vi "NIIE_Check whether installed.vi"(6 "Glyph Name":string, 9 "Glyph Pic":picture, 11 "Glyphs[]":T1[](array[typedef])) -> (1 "Image Out":picture, 2 "Match? Out":bool)   [LabVIEW 2021]
uses:
  MB CORE/TypeDefs/Cluster_Path&Icon.ctl
  vi.lib/LabVIEW Icon API/lv_icon/lv_icon.lvlib
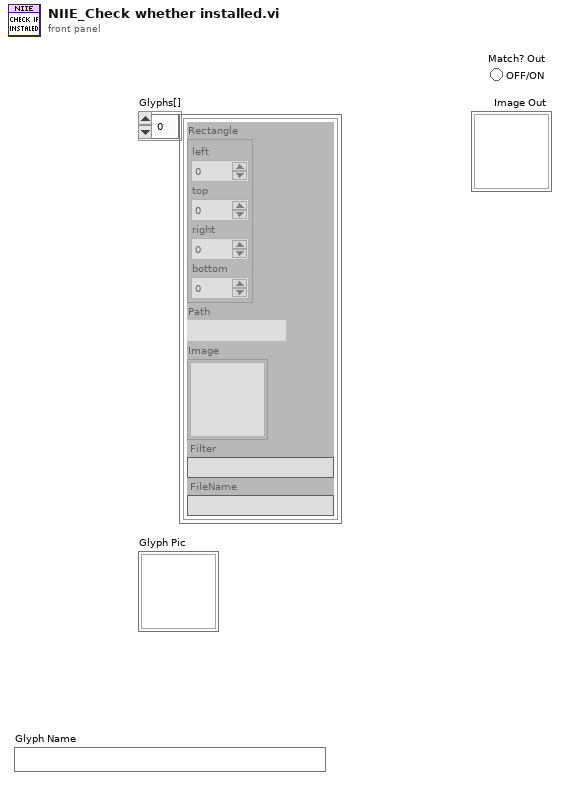
[diagram p1: front panel]
types:
  T1 = typedef "Cluster_Path&Icon.ctl" = cluster{"Rectangle":cluster{"left":i16, "top":i16, "right":i16, "bottom":i16}, "Path":path, "Image":picture, "Filter":string, "FileName":string}
  T2 = typedef "imagedata.ctl" = cluster{"image type":i32, "image depth":i32, "image":u8[], "mask":u8[], "colors":u32[], "Rectangle":cluster{"left":i16, "top":i16, "right":i16, "bottom":i16}}
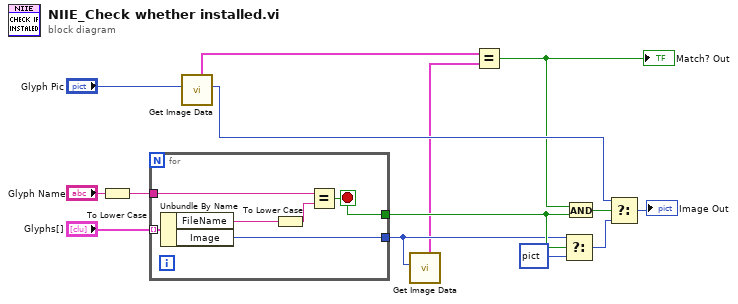
[diagram p0: block diagram]
diagram:
  n1 = To Lower Case(string="Glyph Name") -> (all lower case string=w12:string)
  n2 = for {
    tunnel: "Glyphs[]" -> [w20] mode=indexing
    tunnel: [w19] -> w9
    tunnel: w12 -> [w18]
    tunnel: [w15] -> w4
    stop <- w19 stop-if-true
    n3 = Unbundle By Name(w20) -> ("FileName"=w16:string, "Image"=w15:picture)
    n4 = To Lower Case(string=w16) -> (all lower case string=w17:string)
    n5 = Equal?(x=w18, y=w17) -> (x = y?=w19:bool)
  }
  n6 = call "Get Image Data.vi"("Pic"="Glyph Pic") -> ("Pic Out"=w5:picture, "Image Data Out"=w2:T2)  [unwired: 2 in, 7 out]
  n7 = call "Get Image Data.vi"("Pic"=w4) -> ("Image Data Out"=w1:T2)  [unwired: 2 in, 8 out]
  n8 = Equal?(x=w2, y=w1) -> (x = y?=w3:bool)
  "Match? Out" <- w3
  n9 = Select(t=w4, s=w9, f=picture data[5B]) -> (s? t:f=w7:picture)
  n10 = And(x=w3, y=w9) -> (x .and. y?=w10:bool)
  n11 = Select(t=w5, s=w10, f=w7) -> (s? t:f=→"Image Out":picture)
